vi "Struct Open.vi"(7 "Typedef struct? (F)":bool, 10 "Struct name":string, 11 "String in":string) -> (3 "String out":string)   [LabVIEW 2014, in "C Header Generator.lvlib"]
uses:
  C Header Generator.lvlib
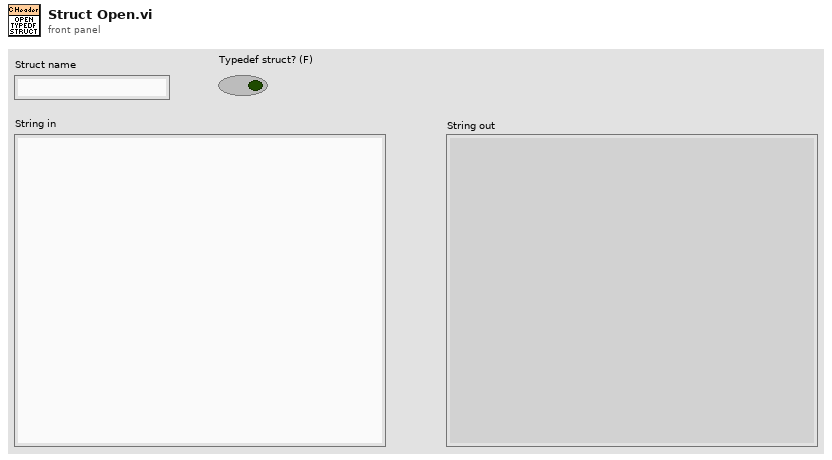
[diagram p1: front panel]
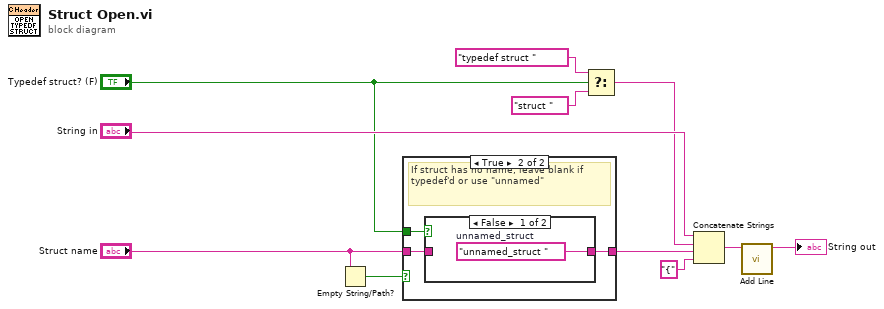
[diagram p0: block diagram]
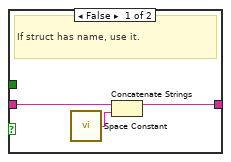
[diagram p2: hidden frame]
diagram:
  n1 = Empty String/Path?(string/path="Struct name") -> (empty?=w2:bool)
  n2 = case shown="True" w2 {
    tunnel: "Struct name" -> [w14 w16]
    tunnel: [w12 w15] -> w10
    tunnel: "Typedef struct? (F)" -> [_ w17]
    frame False {
      # "If struct has name, use it."
      n3 = call <vilib>:"Space Constant.vi"() -> ("String"=w13:string)
      n4 = Concatenate Strings(w14, w13) -> (w12:string)
    }
    frame True {
      # "If struct has no name, leave blank if typedef'd or use \"unnamed\""
      n5 = case shown="False" w17 {
        tunnel: w16 -> [_ w19]
        tunnel: [w18 w19] -> w15
        frame False {
          w18 = "unnamed_struct "  # unnamed_struct
        }
        frame True {
        }
      }
    }
  }
  n6 = Select(t="typedef struct ", s="Typedef struct? (F)", f="struct ") -> (s? t:f=w4:string)
  n7 = Concatenate Strings("String in", w4, w10, "{" ("string")) -> (w8:string)
  n8 = call "Add Line.vi"("String in"=w8) -> ("String out"=→"String out":string)  [unwired: 10 in]
